vi "send abs move to focus stage.vi"(8 "error in (no error)":errorcluster, 10 "absolute position":dbl[unit], 11 "Autofocus in":refnum<class "Autofocus.lvclass">) -> (0 "error out":errorcluster, 3 "Autofocus out":refnum<class "Autofocus.lvclass">)   [LabVIEW 2012, in "Autofocus.lvclass"]
uses:
  Autofocus.lvclass
  <vilib>/Distrio/Murmex/GenericMessage/GenericMessage.lvclass
  <vilib>/Distrio/Murmex/StartMessage/StartMessage.lvclass
  Autofocus.lvclass/Autofocus.ctl
  <vilib>/Distrio/Murmex/Message/Message.lvclass
  <vilib>/Distrio/Murmex/Murmex/Murmex.lvclass
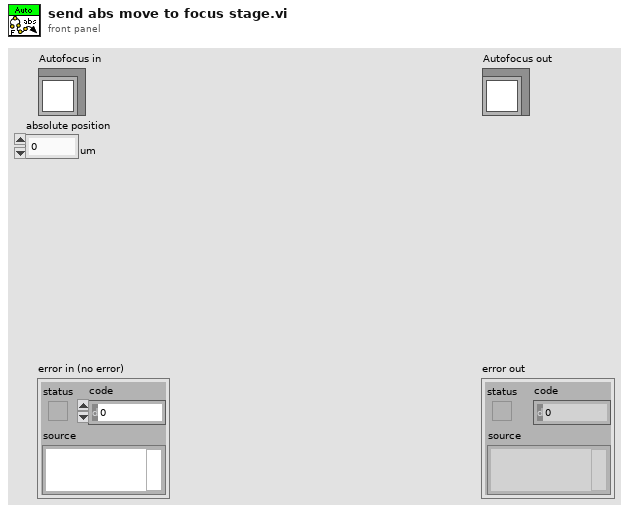
[diagram p1: front panel]
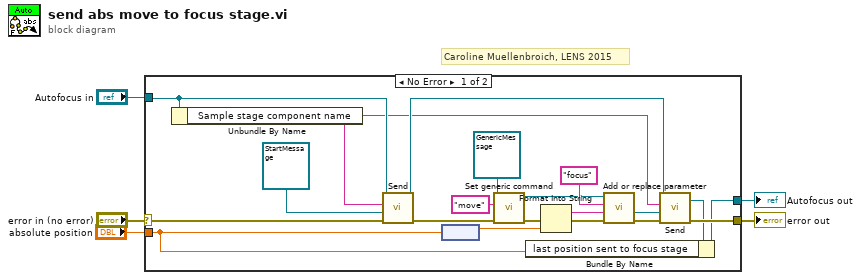
[diagram p0: block diagram]
diagram:
  # "Caroline Muellenbroich, LENS 2015"
  n1 = case shown="No Error" "error in (no error)" {
    selector: "error in (no error)" -> [w11 w27]
    tunnel: [w16 w27] -> w4
    tunnel: [w14 w26] -> w2
    tunnel: "Autofocus in" -> [w9 w26]
    tunnel: "absolute position" -> [w12 _]
    frame No Error {
      n2 = Unbundle By Name(w9) -> ("Sample stage component name"=w7:string)
      n3 = call <vilib>:"Send.vi"("error in (no error)"=w11, "Message"=refnum<class "StartMessage.lvclass"> refnum ("Message in"), "recipient"=w7, "Murmex in"=w9) -> ("error out"=w10:errorcluster, "Murmex out"=w8:refnum<class "Autofocus.lvclass">)  [unwired: 6 in]
      n4 = node(w12) -> (w13:dbl)
      n5 = call <vilib>:"Set generic command.vi"("error in (no error)"=w10, "generic command"="move" ("command string"), "GenericMessage in"=refnum<class "GenericMessage.lvclass"> refnum ("Murmex.lvlib:GenericMessage")) -> ("error out"=w18:errorcluster, "GenericMessage out"=w17:refnum<class "GenericMessage.lvclass">)  [unwired: 7 in]
      n6 = Format Into String(error in=w18, w13) -> (resulting string=w22:string, error out=w21:errorcluster)  [unwired: 2 in]
      n7 = call <vilib>:"Add or replace parameter.vi"("error in (no error)"=w21, "value"=w22, "name"="focus", "Message in"=w17) -> ("error out"=w24:errorcluster, "Message out"=w25:refnum<class "GenericMessage.lvclass">)  [unwired: 6 in]
      n8 = call <vilib>:"Send.vi"("error in (no error)"=w24, "Message"=w25, "recipient"=w7, "Murmex in"=w8) -> ("error out"=w16:errorcluster, "Murmex out"=w15:refnum<class "Autofocus.lvclass">)  [unwired: 6 in]
      n9 = Bundle By Name(cluster=w15, "last position sent to focus stage"=w12) -> (w14:refnum<class "Autofocus.lvclass">)
    }
    frame Error {
    }
  }
  "error out" <- w4
  "Autofocus out" <- w2
